vi "Collect-UI-images.vi"(8 "error in (no error)":errorcluster, 9 "Active display":T1, 10 "Data ref. in":refnum<data-value>, 11 "UI ref. in in":refnum<data-value>) -> (0 "error out":errorcluster, 1 "Image refs":T2[](array[typedef]), 2 "Data ref.":refnum<data-value>, 3 "UI ref. out":refnum<data-value>)   [LabVIEW 2013, in "CameraVision.lvlib" / "CV-UI.lvclass"]
uses:
  CV-UI.lvclass
  Main/CV-Main.lvclass
  <vilib>/vision/Image Controls.llb/IMAQ Image.ctl
  Display-selector.ctl
  CV-UI.lvclass/CV-UI.ctl
  Main/CV-Main.lvclass/CV-Main.ctl
  Main/Read Buffers.vi
  Read Image.vi
  Read Timestep.vi
  Main/Buffers/CV-Buffers.lvclass
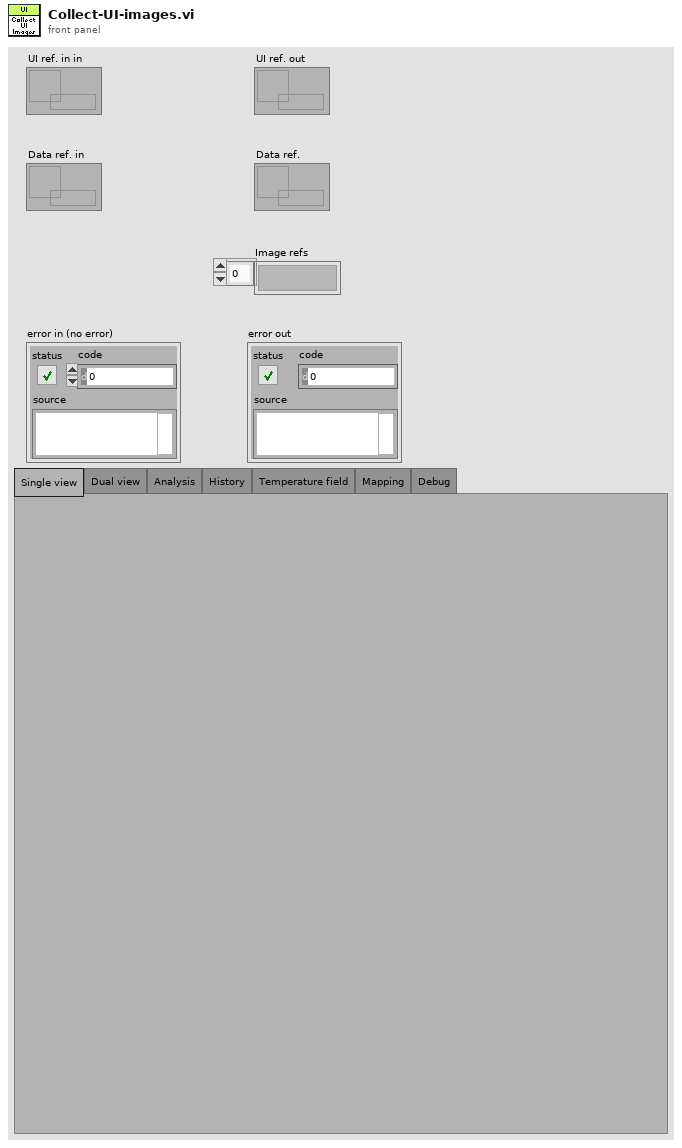
[diagram p1: front panel]
types:
  T1 = typedef "CameraVision.lvlib/CV-UI.lvclass/Display-selector.ctl" = enum32{"Single view", "Dual view", "Analysis", "History", "Temperature field", "Mapping", "Debug"}
  T2 = typedef "IMAQ Image.ctl" = refnum<image>
  T3 = typedef "CameraVision.lvlib/CV-Acquisition.lvclass/Acquisition-stats.ctl" = cluster{"Index":i32, "Time":timestamp, "Acq duration":dbl, "Process duration":dbl}
  T4 = typedef "CameraVision.lvlib/CV-UI.lvclass/Image-selector.ctl" = enum16{"Original", "Corrected", "Binary"}
  T5 = typedef "CameraVision.lvlib/CV-Buffers.lvclass/Storage-buffer-refs.ctl" = cluster{"Raw images":T2[], "Corrected images":T2[], "Binary images":T2[]}
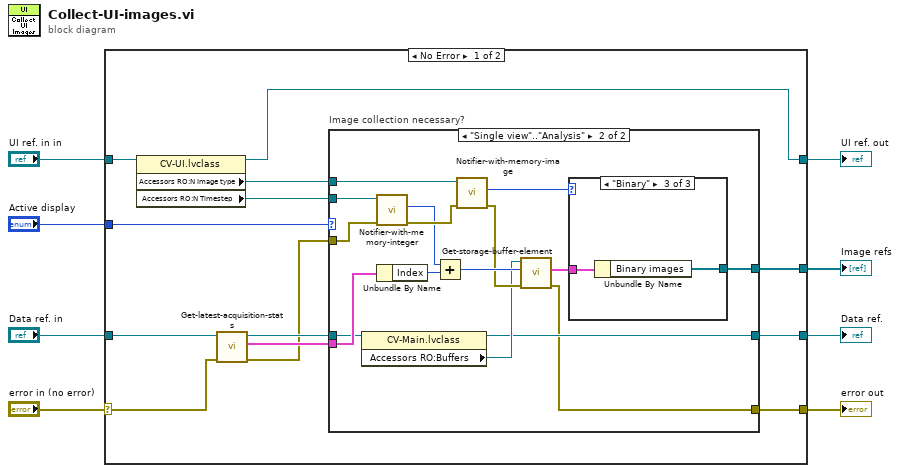
[diagram p0: block diagram]
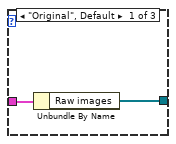
[diagram p3: hidden frame]
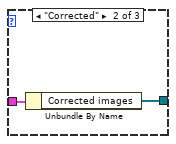
[diagram p4: hidden frame]
diagram:
  n1 = case shown="No Error" "error in (no error)" {
    selector: "error in (no error)" -> [w11 w48]
    tunnel: [w21 w47] -> w8
    tunnel: [w20 _] -> w7
    tunnel: "Data ref. in" -> [w17 w47]
    tunnel: [w16 w48] -> w5
    tunnel: "UI ref. in in" -> [w15 w46]
    tunnel: [w12 w46] -> w3
    tunnel: "Active display" -> [w9 _]
    frame No Error {
      n2 = property class="CV-UI.lvclass"(reference=w15) -> (reference out=w12:refnum<data-value>, "Accessors RO:N Image type"=w14:refnum<notifier>, "Accessors RO:N Timestep"=w13:refnum<notifier>)  [unwired: 1 in, 1 out]
      n3 = call "Get-latest-acquisition-stats.vi"("error in (no error)"=w11, "Data ref. in"=w17) -> ("error out"=w10:errorcluster, "Acq stats"=w18:T3, "Data ref."=w19:refnum<data-value>)  [unwired: 7 in]
      n4 = case "Image collection necessary?" shown="\"Single view\"..\"Analysis\"" w9 {
        tunnel: w13 -> [_ w38]
        tunnel: w10 -> [w23 w39]
        tunnel: [w23 w24] -> w16
        tunnel: w14 -> [_ w37]
        tunnel: w18 -> [_ w35]
        tunnel: w19 -> [w22 w30]
        tunnel: [w22 w26] -> w21
        tunnel: [_ w25] -> w20
        frame Default {
        }
        frame "Single view".."Analysis" {
          n5 = property class="CV-Main.lvclass"(reference=w30) -> (reference out=w26:refnum<data-value>, "Accessors RO:Buffers"=w29:refnum<class "CV-Buffers.lvclass">)  [unwired: 1 in, 1 out]
          n6 = call "Notifier-with-memory-integer.vi"("error in"=w39, "Notifier in"=w38) -> ("error IO"=w36:errorcluster, "Notification"=w33:i32)  [unwired: 8 in]
          n7 = Unbundle By Name(w35) -> ("Index"=w34:i32)
          n8 = Add(x=w33, y=w34) -> (x+y=w32:i32)
          n9 = call "Notifier-with-memory-image.vi"("error in"=w36, "Notifier in"=w37) -> ("error IO"=w31:errorcluster, "Notification"=w27:T4)  [unwired: 8 in]
          n10 = call "Get-storage-buffer-element.vi"("error in (no error)"=w31, "Index"=w32, "Buffers in"=w29) -> ("error out"=w24:errorcluster, "Element ref"=w28:T5)  [unwired: 6 in, 1 out]
          n11 = case shown="\"Binary\"" w27 {
            tunnel: w28 -> [w41 w43 w45]
            tunnel: [w40 w42 w44] -> w25
            frame "Original", Default {
              n12 = Unbundle By Name(w41) -> ("Raw images"=w40:T2[])
            }
            frame "Corrected" {
              n13 = Unbundle By Name(w43) -> ("Corrected images"=w42:T2[])
            }
            frame "Binary" {
              n14 = Unbundle By Name(w45) -> ("Binary images"=w44:T2[])
            }
          }
        }
      }
    }
    frame Error {
    }
  }
  "UI ref. out" <- w3
  "Data ref." <- w8
  "Image refs" <- w7
  "error out" <- w5
